vi "Simple Error Out Facade.vi"(0 "Data In":T4, 2 "Display State In":T2, 3 "Container State":T3) -> (6 "Data Out":T4, 7 "Display State Out":T2, 8 "Action":T1)   [LabVIEW 2011, in "Simple Error Out.xctl"]
uses:
  Simple Error Out.xctl
  Simple Error Out Data.ctl
  <vilib>/_xctls/Container State.ctl
  Simple Error Out State.ctl
  <vilib>/_xctls/Action.ctl
  <vilib>/_xctls/XControlSupport.lvlib
panel:
  out "Type":enum16{"None", "Warning", "Error"}(ring)
  out "error out":bool=TRUE
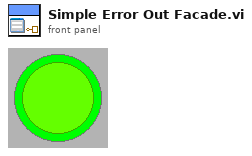
[diagram p1: front panel]
types:
  T1 = typedef "XControlSupport.lvlib/Action.ctl" = cluster{"Data Changed?":bool, "State Changed?":bool, "Action Name":string}
  T2 = typedef "Simple Error Out.xctl/Simple Error Out State.ctl" = cluster{"Numeric":dbl}
  T3 = typedef "XControlSupport.lvlib/Container State.ctl" = cluster{"Indicator?":bool, "Run Mode?":bool, " Refnum":refnum<vi>}
  T4 = typedef "Simple Error Out.xctl/Simple Error Out Data.ctl" = errorcluster
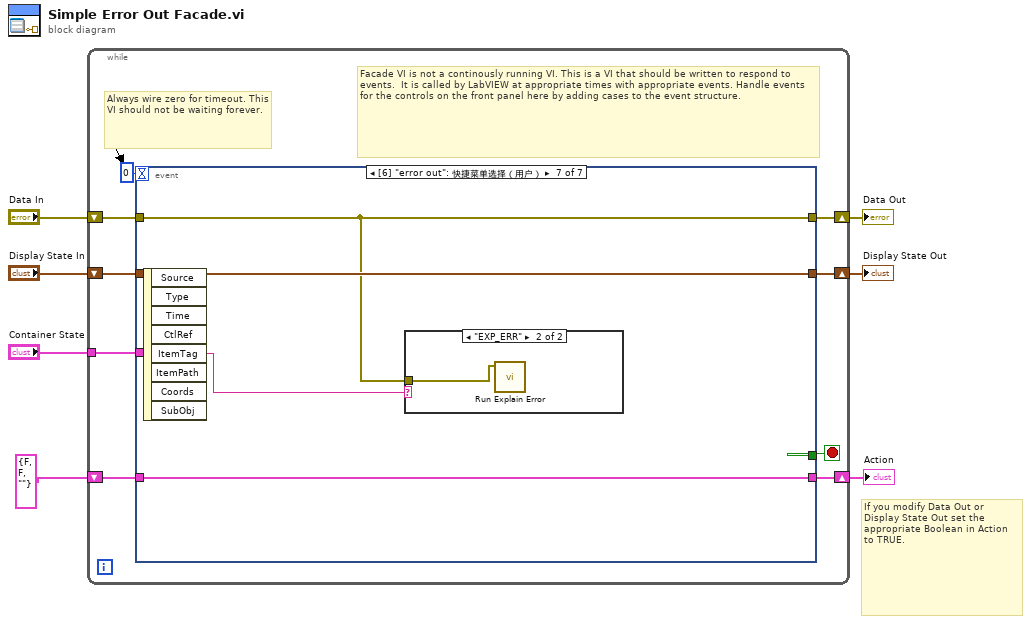
[diagram p0: block diagram]
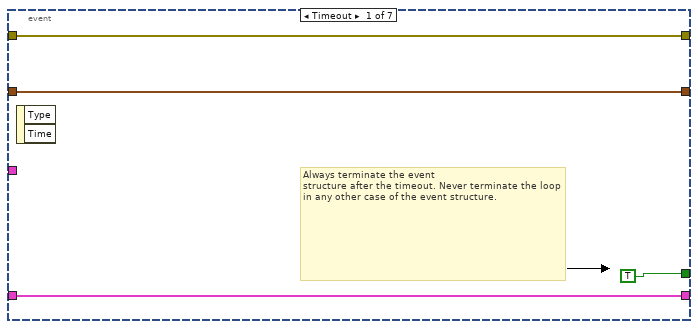
[diagram p2: hidden frame]
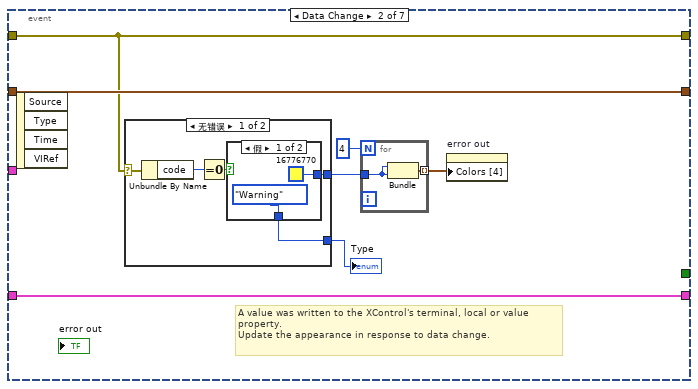
[diagram p3: hidden frame]
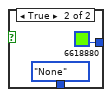
[diagram p4: hidden frame]
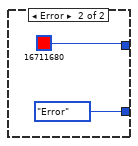
[diagram p5: hidden frame]
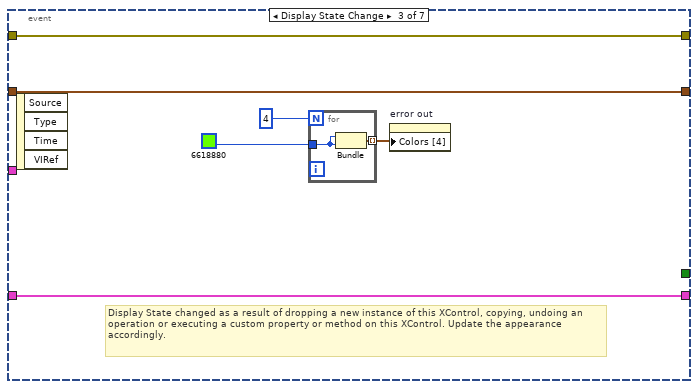
[diagram p6: hidden frame]
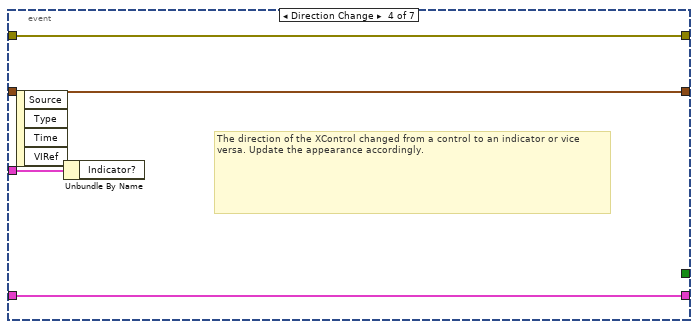
[diagram p7: hidden frame]
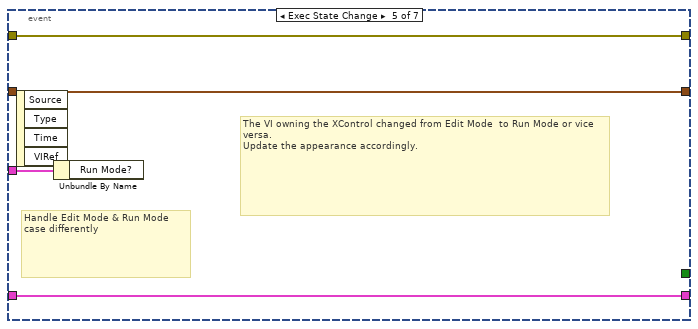
[diagram p8: hidden frame]
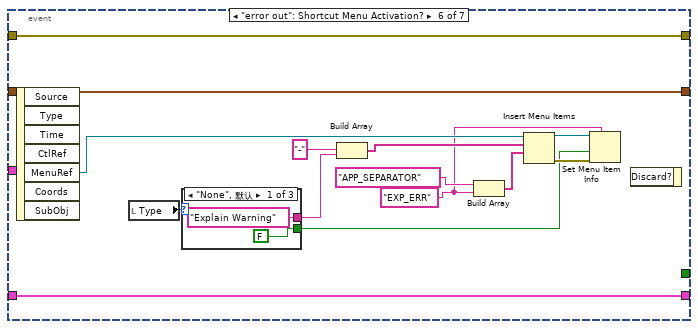
[diagram p9: hidden frame]
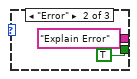
[diagram p10: hidden frame]
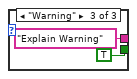
[diagram p11: hidden frame]
diagram:
  # "If you modify Data Out or\nDisplay State Out set the\nappropriate Boolean in Action\nto TRUE."
  n1 = while {
    shift-right: [w15] -> w4
    shift-left: "Display State In" -> [w16]
    tunnel: "Container State" -> [w12]
    shift-right: [w10] -> w7
    shift-left: "Data In" -> [w11]
    shift-right: [w8] -> w2
    shift-left: T1 {"Data Changed?"=FALSE, "State Changed?"=FALSE, "Action Name"=""} ("Action") -> [w9]
    stop <- w14 stop-if-true
    # "Facade VI is not a continously running VI. This is a VI that should be written to respond to events.  It is called by LabVIEW at appropriate times with appropriate events. Handle events for the controls on the front panel here by adding cases to the event structure."
    # "Always wire zero for timeout. This\nVI should not be waiting forever."
    n2 = event shown="[6] \"error out\": 快捷菜单选择（用户）" {
      selector: _ -> [_ _ _ _ _ _ _]
      dyn-events: _ -> [_ _ _ _ _ _ _]
      timeout: 0 -> [_ _ _ _ _ _ _]
      tunnel: w16 -> [w18 w27 w46 w51 w55 w69 w80]
      tunnel: [w18 w27 w46 w51 w55 w69 w80] -> w15
      tunnel: [TRUE _ _ _ _ _ _] -> w14
      tunnel: w12 -> [_ _ _ w52 w56 _ _]
      tunnel: w11 -> [w17 w24 w45 w50 w54 w70 w77]
      tunnel: [w17 w24 w45 w50 w54 w70 w77] -> w10
      tunnel: [w19 w26 w44 w49 w53 w68 w79] -> w8
      tunnel: w9 -> [w19 w26 w44 w49 w53 w68 w79]
      event Timeout {
        # "Always terminate the event\nstructure after the timeout. Never terminate the loop in any other case of the event structure."
        n3 = event-data() -> ()  [unwired: 1 in, 2 out]
      }
      event Data Change {
        # "A value was written to the XControl's terminal, local or value property.\nUpdate the appearance in response to data change."
        n4 = event-data() -> ()  [unwired: 1 in, 4 out]
        n5 = case shown="无错误" w24 {
          selector: w24 -> [w32 _]
          tunnel: [w29 u32 16711680] -> w23
          tunnel: [w28 enum16{"None", "Warning", "Error"}."Error" ("Type")] -> w21
          frame No Error {
            n6 = Unbundle By Name(w32) -> ("code"=w30:i32)
            n7 = Equal To 0?(x=w30) -> (x = 0?=w31:bool)
            n8 = case shown="假" w31 {
              tunnel: [u32 16776770 u32 6618880] -> w29
              tunnel: [enum16{"None", "Warning", "Error"}."Warning" ("Type") enum16{"None", "Warning", "Error"}."None" ("Type")] -> w28
              frame False {
              }
              frame True {
              }
            }
          }
          frame Error {
          }
        }
        "Type" <- w21
        n9 = for {
          N: 4 -> [_]
          tunnel: w23 -> [w40]
          tunnel: [w39] -> w22 mode=indexing
          n10 = Bundle(w40, w40) -> (w39:cluster{u32, u32})  [unwired: 1 in]
        }
        n11 = property on="error out" class="Bool (严格)"("Colors [4]"=w22) -> ()  [unwired: 2 in, 2 out]
      }
      event Display State Change {
        # "Display State changed as a result of dropping a new instance of this XControl, copying, undoing an operation or executing a custom property or method on this XControl. Update the appearance accordingly."
        n12 = event-data() -> ()  [unwired: 1 in, 4 out]
        n13 = for {
          N: 4 -> [_]
          tunnel: u32 6618880 -> [w48]
          tunnel: [w47] -> w42 mode=indexing
          n14 = Bundle(w48, w48) -> (w47:cluster{u32, u32})  [unwired: 1 in]
        }
        n15 = property on="error out" class="Bool (严格)"("Colors [4]"=w42) -> ()  [unwired: 2 in, 2 out]
      }
      event Direction Change {
        # "The direction of the XControl changed from a control to an indicator or vice versa. Update the appearance accordingly."
        n16 = event-data() -> ()  [unwired: 1 in, 4 out]
        n17 = Unbundle By Name(w52) -> ()  [unwired: 1 out]
      }
      event Exec State Change {
        # "The VI owning the XControl changed from Edit Mode  to Run Mode or vice versa.\nUpdate the appearance accordingly."
        # "Handle Edit Mode & Run Mode\ncase differently"
        n18 = event-data() -> ()  [unwired: 1 in, 4 out]
        n19 = Unbundle By Name(w56) -> ()  [unwired: 1 out]
      }
      event "error out": Shortcut Menu Activation? {
        w58 = "EXP_ERR" ("element")
        n20 = event-data() -> ("MenuRef"=w62:refnum<k9>)  [unwired: 1 in, 6 out]
        n21 = local read "Type"() -> (w61:enum16{"None", "Warning", "Error"})
        n22 = case shown="\"None\", 默认" w61 {
          tunnel: ["Explain Warning" ("Item Name") "Explain Error" ("Item Name") "Explain Warning" ("Item Name")] -> w66
          tunnel: [FALSE TRUE TRUE] -> w57
          frame "None", Default {
          }
          frame "Error" {
          }
          frame "Warning" {
          }
        }
        n23 = Build Array("-", w66) -> (w65:string[])
        n24 = Build Array("APP_SEPARATOR", w58) -> (w64:string[])
        n25 = Insert Menu Items(7:w64, 8:w65, 9:w62) -> (0:w60:errorcluster, 3:w59:refnum<k9>)  [unwired: 3 in, 1 out]
        n26 = Set Menu Item Info(7:w58, 8:w60, 9:w57, 11:w59) -> ()  [unwired: 3 in, 2 out]
        n27 = event-data() -> ()  [unwired: 2 in, 1 out]
      }
      event "error out": Shortcut Menu Selection (User) {
        n28 = event-data() -> ("ItemTag"=w78:string)  [unwired: 1 in, 7 out]
        n29 = case shown="\"EXP_ERR\"" w78 {
          tunnel: w77 -> [_ w81]
          frame Default {
          }
          frame "EXP_ERR" {
            n30 = call "Run Explain Error.vi"("Data"=w81) -> ()  [unwired: 10 in, 1 out]
          }
        }
      }
    }
  }
  "Display State Out" <- w4
  "Data Out" <- w7
  "Action" <- w2
